vi "Create DatabaseTable.vi"() -> ()   [LabVIEW 2012]
doc: "This example allows you to perform several tasks on a database named LabVIEW.mdb located in the LabVIEW examples>>database directory.\n\nOperations include creating a table, creating a table and inserting data into named fields, creating a table and inserting data into generically named fields, or deleting a table."
uses:
  Connection.llb/DB Tools Open Connec (Path).vi
  NI_Database_API_64.lvlib
  Auxilliary.llb/DB Tools DataTypes.ctl
  Auxilliary.llb/DB Tools Column Info.ctl
panel:
  in  "sample data":T1={"String"="This is a test string", "Numeric"=101, "Numeric 2"=3.14} {"Numeric 2" format="%.2f"}
  in  "column information":T2[](array[typedef])=[{"column name"="stringcol", "data type"=enum."String", "size"=50, "allow null?"=FALSE}, {"column name"="intcol", "data type"=enum."Long (I32)", "size"=0, "allow null?"=TRUE}, {"column name"="doublecol", "data type"=enum."Double (DBL)", "size"=0, "allow null?"=TRUE}]
  in  "Function":T4(ring)
  in  "Table":string="createtable"
  # "INSTRUCTIONS:\n\nChoose which method to use to create the table by clicking an option in the Function ring.  Run the VI.  You do not have to change any of the data in the controls as they are already correctly set up."
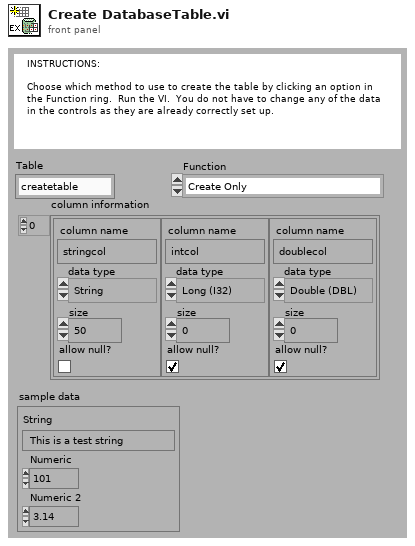
[diagram p1: front panel]
types:
  T1 = cluster{"String":string, "Numeric":i32, "Numeric 2":dbl}
  T2 = typedef "NI_Database_API_64.lvlib/DB Tools Column Info.ctl" = cluster{"column name":string, "data type":T3, "size":i32, "allow null?":bool}
  T3 = typedef "NI_Database_API_64.lvlib/DB Tools DataTypes.ctl" = enum16{"String", "Long (I32)", "Single (SGL)", "Double (DBL)", "Date/Time", "Binary"}
  T4 = enum16{"Create Only", "Create & Insert (with Names)", "Create & Insert (Generic Names)", "Delete Table"}
  T5 = typedef "NI_Database_API_64.lvlib/Conn ObjectReference.ctl" = refnum<k1>
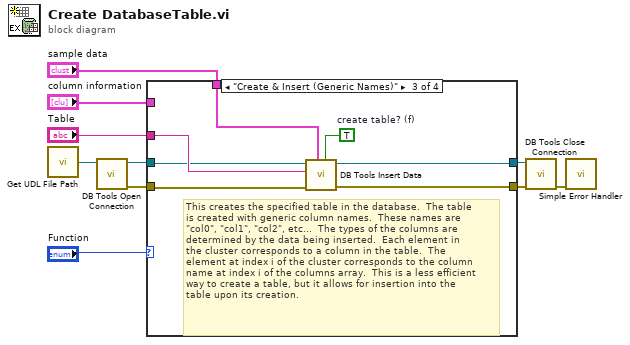
[diagram p0: block diagram]
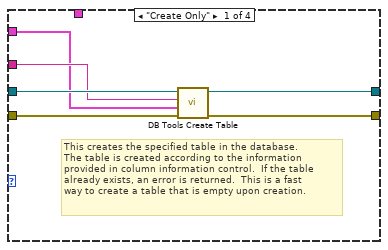
[diagram p2: hidden frame]
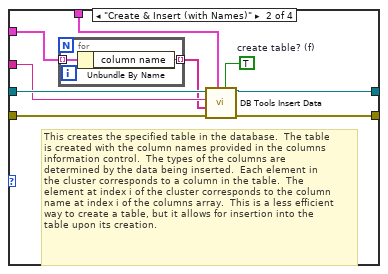
[diagram p3: hidden frame]
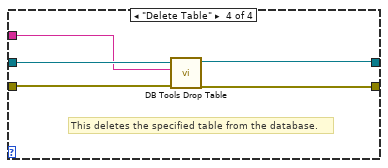
[diagram p4: hidden frame]
diagram:
  n1 = call "Get UDL File Path.vi"() -> ("UDL file path"=w10:path)  [unwired: 1 in]
  n2 = call-poly "DB Tools Open Connection.vi"("connection information"=w10) -> ("error out"=w5:errorcluster, "connection reference"=w6:T5)  [unwired: 7 in]
  n3 = case shown="\"Create & Insert (Generic Names)\"" "Function" {
    tunnel: w6 -> [w16 w25 w29 w39]
    tunnel: w5 -> [w15 w22 w30 w38]
    tunnel: "Table" -> [w14 w19 w31 w35]
    tunnel: [w13 w20 w32 w37] -> w8
    tunnel: [w12 w21 w34 w36] -> w7
    tunnel: "sample data" -> [_ w23 w28 _]
    tunnel: "column information" -> [w11 w18 _ _]
    frame "Create Only" {
      # "This creates the specified table in the database. \nThe table is created according to the information \nprovided in column information control.  If the table \nalready exists, an error is returned.  This is a fast \nway to create a table that is empty upon creation."
      n4 = call "DB Tools Create Table.vi"("error in (no error)"=w15, "column information"=w11, "table"=w14, "connection reference"=w16) -> ("error out"=w12:errorcluster, "connection reference out"=w13:T5)  [unwired: 4 in]
    }
    frame "Create & Insert (with Names)" {
      w24 = TRUE  # create table? (f)
      # "This creates the specified table in the database.  The table \nis created with the column names provided in the columns \ninformation control.  The types of the columns are \ndetermined by the data being inserted.  Each element in \nthe cluster corresponds to a column in the table.  The \nelement at index i of the cluster corresponds to the column \nname at index i of the columns array.  This is a less efficient \nway to create a table, but it allows for insertion into the \ntable upon its creation."
      n5 = for {
        tunnel: w18 -> [w27] mode=indexing
        tunnel: [w26] -> w17 mode=indexing
        n6 = Unbundle By Name(w27) -> ("column name"=w26:string)
      }
      n7 = call "DB Tools Insert Data.vi"("create table? (F)"=w24, "data"=w23, "error in (no error)"=w22, "columns"=w17, "table"=w19, "connection reference"=w25) -> ("error out"=w21:errorcluster, "connection reference out"=w20:T5)  [unwired: 4 in]
    }
    frame "Create & Insert (Generic Names)" {
      w33 = TRUE  # create table? (f)
      # "This creates the specified table in the database.  The table \nis created with generic column names.  These names are \n\"col0\", \"col1\", \"col2\", etc...  The types of the columns are\ndetermined by the data being inserted.  Each element in \nthe cluster corresponds to a column in the table.  The \nelement at index i of the cluster corresponds to the column \nname at index i of the columns array.  This is a less efficient \nway to create a table, but it allows for insertion into the \ntable upon its creation."
      n8 = call "DB Tools Insert Data.vi"("create table? (F)"=w33, "data"=w28, "error in (no error)"=w30, "table"=w31, "connection reference"=w29) -> ("error out"=w34:errorcluster, "connection reference out"=w32:T5)  [unwired: 5 in]
    }
    frame "Delete Table" {
      # "This deletes the specified table from the database."
      n9 = call "DB Tools Drop Table.vi"("error in (no error)"=w38, "table"=w35, "connection reference"=w39) -> ("error out"=w36:errorcluster, "connection reference out"=w37:T5)  [unwired: 5 in]
    }
  }
  n10 = call "DB Tools Close Connection.vi"("error in (no error)"=w7, "connection reference"=w8) -> ("error out"=w3:errorcluster)  [unwired: 5 in]
  n11 = call <vilib>:"Simple Error Handler.vi"("error in (no error)"=w3) -> ()  [unwired: 4 in, 5 out]
